vi "Abort-plant.vi"(8 "error in (no error)":errorcluster, 10 "Plant VI path":path=path "C:/ni-rt/startup/Plant1.vi") -> (0 "error out":errorcluster)   [LabVIEW 2016]
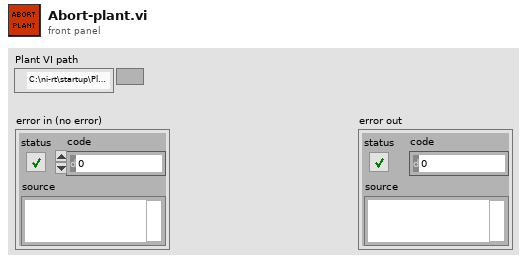
[diagram p1: front panel]
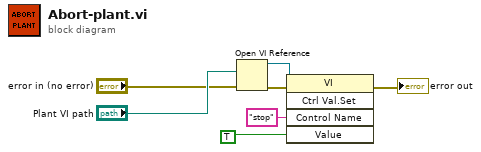
[diagram p0: block diagram]
diagram:
  n1 = Open VI Reference(vi path="Plant VI path", error in (no error)="error in (no error)") -> (vi reference=w6:refnum<vi>, error out=w5:errorcluster)  [unwired: 4 in]
  n2 = invoke class="VI" method="Ctrl Val.Set"(reference=w6, error in=w5, "Control Name"="stop", "Value"=TRUE) -> (error out=→"error out":errorcluster)  [unwired: 1 in, 4 out]
